vi "PerformDAQ.vi"(0 "PM Cmds In":refnum<k24>, 5 "Device Key In":string, 7 "Interval":string, 9 "Sample Size":string, 11 "error in":errorcluster) -> (4 "PM Cmds Out":refnum<k24>, 6 "Device Key Out":string, 8 "Data Acquisition":dbl[](array[numeric]), 15 "error out":errorcluster)   [LabVIEW 2009]
uses:
  C:/Code/Apps/Utilities/PM2935/PMWinApp/PM_Installer/Master/Samples/1918 - 2936 Family/LabVIEW/LabVIEW 2009/PowerMeterCommands.dll
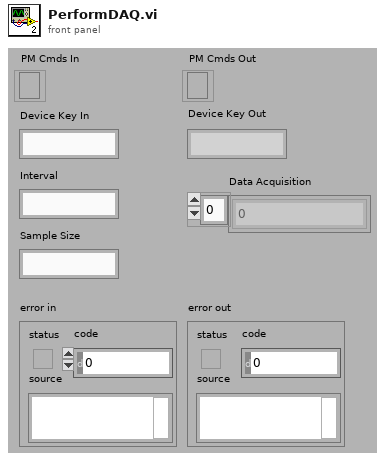
[diagram p1: front panel]
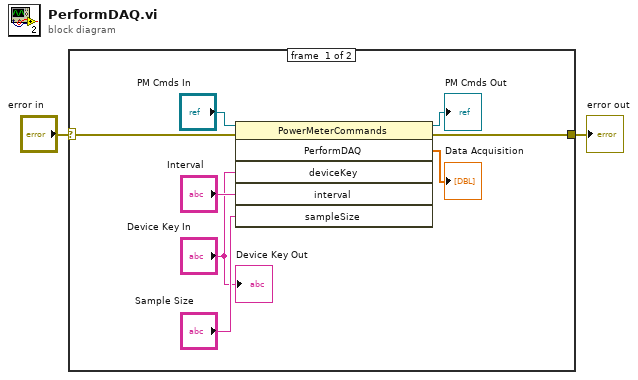
[diagram p0: block diagram]
diagram:
  n1 = case shown="No Error" "error in" {
    selector: "error in" -> [w5 w11]
    tunnel: [w10 w11] -> w2
    frame #0 {
      n2 = invoke class="PowerMeterCommands" method="PerformDAQ"(reference="PM Cmds In", error in=w5, "deviceKey"="Device Key In", "interval"="Interval", "sampleSize"="Sample Size") -> (reference out=→"PM Cmds Out":refnum<k24>, error out=w10:errorcluster, "PerformDAQ"=→"Data Acquisition":dbl[])  [unwired: 1 in, 3 out]
      "Device Key Out" <- "Device Key In"
    }
    frame #1 {
    }
  }
  "error out" <- w2
